vi "templates standard HEADER data keys.vi"(9 "Template Keys":T1, 10 "HTM Keys":T1) -> (2 "HTM Keys":T1)   [LabVIEW 2011]
uses:
  Addons/internet/utils/keyedarr.llb/Keyed Array.ctl
  Addons/internet/utils/strutil.llb/Case Matching.ctl
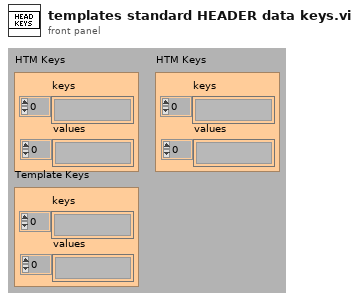
[diagram p1: front panel]
types:
  T1 = typedef "Keyed Array.ctl" = cluster{"keys":string[], "values":string[]}
  T2 = typedef "Case Matching.ctl" = enum16{"a != A", "a == A", "system"}
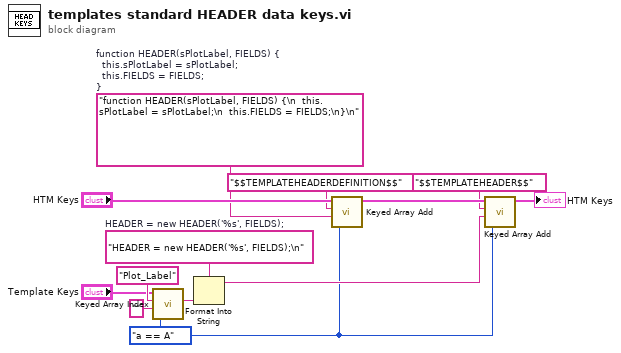
[diagram p0: block diagram]
diagram:
  w1 = Case_Matching."a == A" ("case matching (sensitive)")
  w4 = "HEADER = new HEADER('%s', FIELDS);\n"  # HEADER = new HEADER('%s', FIELDS);
  w11 = "function HEADER(sPlotLabel, FIELDS) {\n  this.sPlotLabel = sPlotLabel;\n  this.FIELDS = FIELDS;\n}\n"  # function HEADER(sPlotLabel, FIELDS) {   this.sPlotLabel = sPlotLabel;   this.FIELDS = FIELDS; }
  n1 = call "Keyed Array Index.vi"("case matching (sensitive)"=w1, "default value"="" ("key"), "key"="Plot_Label", "array in"="Template Keys") -> ("value"=w2:string)  [unwired: 3 out]
  n2 = Format Into String(format string=w4, w2) -> (resulting string=w3:string)  [unwired: 2 in, 1 out]
  n3 = call "Keyed Array Add.vi"("case matching (sensitive)"=w1, "value"=w11, "key"="$$TEMPLATEHEADERDEFINITION$$", "array in"="HTM Keys") -> ("array out"=w10:T1)  [unwired: 3 out]
  n4 = call "Keyed Array Add.vi"("case matching (sensitive)"=w1, "value"=w3, "key"="$$TEMPLATEHEADER$$", "array in"=w10) -> ("array out"=→"HTM Keys":T1)  [unwired: 3 out]
